vi "CC Focus Generate Focus Scan Script.vi"(7 "Images":i32=10, 8 "error in (no error)":errorcluster, 9 "Exp Time":dbl format="%.1g", 10 "Motor 0 Steps":i32, 11 "Motor 1 Steps":i32) -> (0 "error out":errorcluster, 3 "Script":T1[](array[typedef]))   [LabVIEW 2024]
uses:
  typedefs/CC Script Step.ctl
  typedefs/CC enum Script Action.ctl
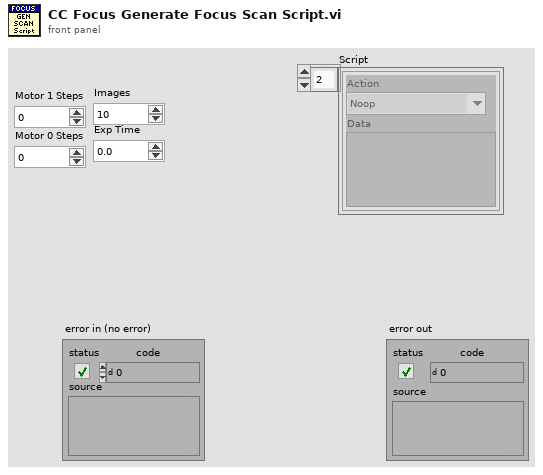
[diagram p1: front panel]
types:
  T1 = typedef "CC Script Step.ctl" = cluster{"Action":T2, "Data":variant}
  T2 = typedef "CC enum Script Action.ctl" = enum16{"Noop", "Define Object", "Define Exposure", "Define Dithering", "Acquire Images", "Set Filter Wheel", "Telescope Home", "Telescope Move", "Telescope RA DEC", "Focus Move Relative", "Focus Move Absolute", "Focus Set Home", "Macro", "Pause", "Ask User", "Define Random Dither", "CmdLine", "Outlet"}
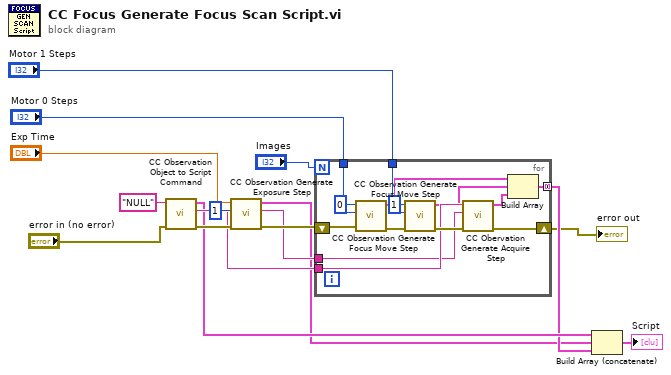
[diagram p0: block diagram]
diagram:
  n1 = call "CC Observation Object to Script Command.vi"("error in (no error)"="error in (no error)", "Object.Name"="NULL") -> ("error out"=w13:errorcluster, "Object Name out"=w9:string, "Define Object Step"=w7:T1)  [unwired: 7 in]
  n2 = call "CC Observation Generate Exposure Step.vi"("error in (no error)"=w13, "Images"=1, "Integration Time"="Exp Time") -> ("error out"=w10:errorcluster, "Exp Name"=w8:string, "Exp Step"=w4:T1)  [unwired: 6 in]
  n3 = for {
    N: "Images" -> [_]
    tunnel: "Motor 0 Steps" -> [w30]
    tunnel: "Motor 1 Steps" -> [w29]
    tunnel: w9 -> [w23]
    tunnel: w8 -> [w22]
    tunnel: [w18] -> w5 mode=concatenating
    shift-right: [w17] -> w2
    shift-left: w10 -> [w26]
    n4 = call "CC Observation Generate Focus Move Step.vi"("error in (no error)"=w26, "Position"=w30, "Motor"=0) -> ("error out"=w25:errorcluster, "Exp Step"=w21:T1)  [unwired: 7 in]
    n5 = call "CC Observation Generate Focus Move Step.vi"("error in (no error)"=w25, "Position"=w29, "Motor"=1) -> ("error out"=w24:errorcluster, "Exp Step"=w20:T1)  [unwired: 7 in]
    n6 = call "CC Obervation Generate Acquire Step.vi"("error in (no error)"=w24, "Exposure"=w22, "Object"=w23) -> ("error out"=w17:errorcluster, "Acquire Step"=w19:T1)  [unwired: 7 in]
    n7 = Build Array(w21, w20, w19) -> (w18:T1[])
  }
  "error out" <- w2
  n8 = Build Array (concatenate)(w7, w4, w5) -> (→"Script":T1[])
